vi "Run 01.vi"   [LabVIEW 2016]
types:
  T1 = typedef "LVHSConnector.ctl" = refnum<class "BrickReference.lvclass">
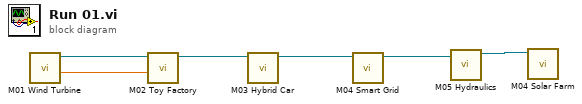
[diagram p0: block diagram]
diagram:
  n1 = call "M01 Wind Turbine.vi"() -> ("Angle out"=w5:sgl, "EV3 out"=w6:T1)  [unwired: 10 in]
  n2 = call "M02 Toy Factory.vi"("Angle in"=w5, "EV3 in"=w6) -> ("EV3 out"=w4:T1)  [unwired: 9 in]
  n3 = call "M03 Hybrid Car.vi"("EV3 in"=w4) -> ("EV3 out"=w3:T1)  [unwired: 10 in]
  n4 = call "M04 Smart Grid.vi"("EV3 in"=w3) -> ("EV3 out"=w2:T1)  [unwired: 10 in]
  n5 = call "M05 Hydraulics.vi"("NXT/EV3"=w2) -> ("NXT/EV3 2"=w1:T1)  [unwired: 10 in]
  n6 = call "M04 Solar Farm.vi"("EV3 in"=w1) -> ()  [unwired: 11 in]
